vi "cRIO Memory Perc Calc.vi"(8 "error in (no error)":errorcluster, 9 "error IO in":errorcluster, 10 "Memory Total (bytes)":u32, 11 "Memory Used (bytes)":u32) -> (0 "error out":errorcluster, 3 "Memory Used (%)":dbl)   [LabVIEW 2016, in "Top Level.lvlib"]
uses:
  Top level/Top Level.lvlib
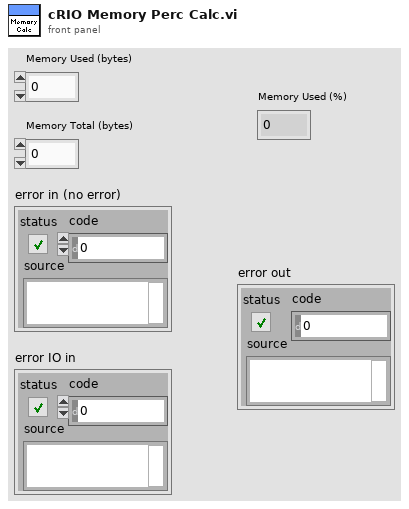
[diagram p1: front panel]
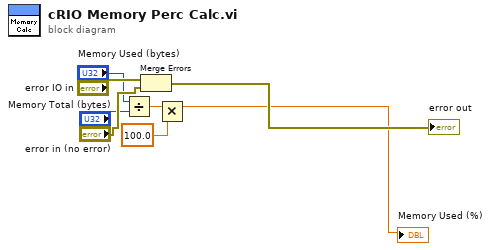
[diagram p0: block diagram]
diagram:
  n1 = Divide(x="Memory Used (bytes)", y="Memory Total (bytes)") -> (x/y=w3:dbl)
  n2 = Merge Errors("error IO in", "error in (no error)") -> (→"error out":errorcluster)
  n3 = Multiply(x=w3, y=100.0) -> (x*y=→"Memory Used (%)":dbl)
